vi "Servo MSMT Get Measure Step from DB.vi"(8 "error in (no error)":errorcluster, 10 "Standard":string, 11 "Servo MSMT in":refnum<class "Servo MSMT.lvclass">) -> (0 "error out":errorcluster, 2 "Step Out":refnum<k7>, 3 "Servo MSMT out":refnum<class "Servo MSMT.lvclass">)   [LabVIEW 2018, in "Servo MSMT.lvlib" / "Servo MSMT.lvclass"]
uses:
  Servo MSMT.lvclass
  C:/Sequence Automation/Plugins/Measurement Interface.lvlibp/Measurement Interface.lvclass
  Plugins/Measurement Interface.lvlibp/Private Methods/Measurement Name/Read Measurement Name.vi
  Plugins/TestStand API Tools (TSAT).lvlibp/Step Actions/TSAT Step Actions.lvlib
  Plugins/Measurement Interface.lvlibp/Measurement Interface.lvclass
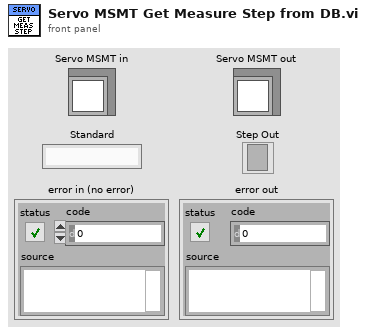
[diagram p1: front panel]
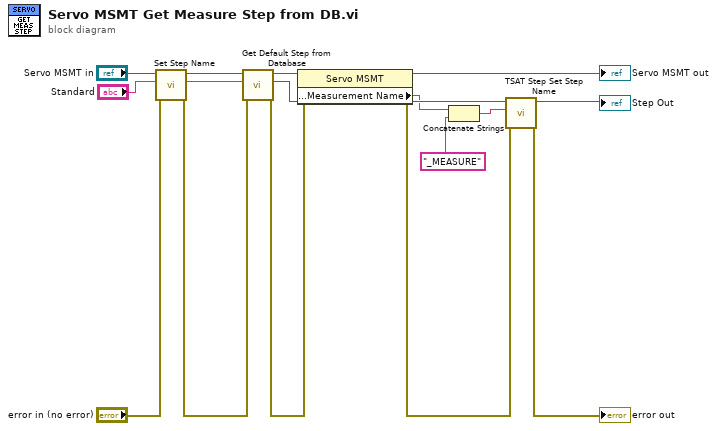
[diagram p0: block diagram]
diagram:
  n1 = call-dynamic "Set Step Name.vi"("error in (no error)"="error in (no error)", "Standard"="Standard", "Servo MSMT in"="Servo MSMT in") -> ("error out"=w15:errorcluster, "Default Step"=w12:string, "Servo MSMT out"=w13:refnum<class "Servo MSMT.lvclass">)  [unwired: 6 in]
  n2 = call "Get Default Step from Database.vi"("error in (no error)"=w15, "Default Step"=w12, "Measurement Interface in"=w13) -> ("error out"=w8:errorcluster, "Cloned Step"=w11:refnum<k7>, "Measurement Interface out"=w5:refnum<class "Servo MSMT.lvclass">)  [unwired: 6 in]
  n3 = property class="Servo MSMT"(reference=w5, error in=w8) -> (reference out=→"Servo MSMT out":refnum<class "Servo MSMT.lvclass">, error out=w6:errorcluster, "Public Methods:Measurement Name"=w3:string)
  n4 = Concatenate Strings(w3, "_MEASURE" ("string")) -> (w2:string)
  n5 = call "TSAT Step Set Step Name.vi"("Error In"=w6, "Name"=w2, "Step In"=w11) -> ("Error Out"=→"error out":errorcluster, "Step Out"=→"Step Out":refnum<k7>)  [unwired: 7 in]
